vi "TreeMenuUpdate.vi"(4 "error in":errorcluster, 5 "Date?":bool, 6 "stripped path":path, 7 "Tree Refnum":refnum<vi>) -> (0 "error out":errorcluster)   [LabVIEW 2013, in "main.lvlib"]
uses:
  main.lvlib
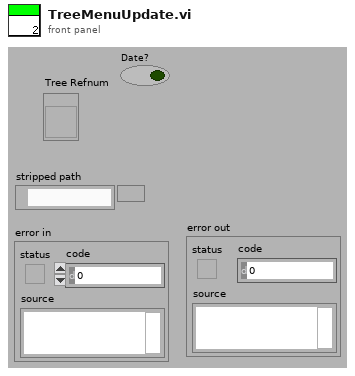
[diagram p1: front panel]
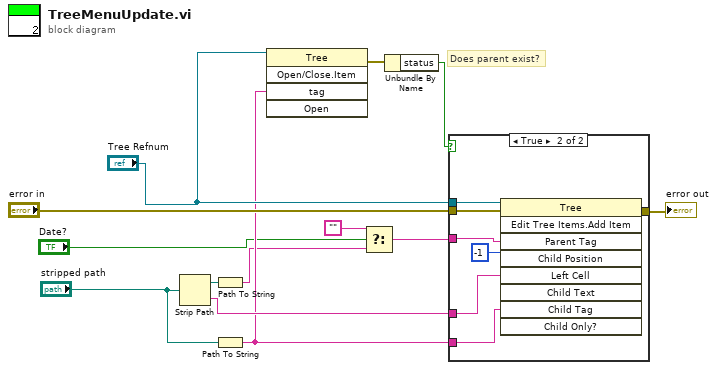
[diagram p0: block diagram]
diagram:
  # "Does parent exist?"
  n1 = Strip Path(path="stripped path") -> (stripped path=w9:path, name=w12:string)
  n2 = Path To String(path=w9) -> (string=w4:string)
  n3 = Path To String(path="stripped path") -> (string=w5:string)
  n4 = invoke class="Tree" method="Open/Close.Item"(reference="Tree Refnum", "tag"=w5) -> (error out=w7:errorcluster)  [unwired: 3 in, 4 out]
  n5 = Select(t="", s="Date?", f=w4) -> (s? t:f=w1:string)
  n6 = Unbundle By Name(w7) -> ("status"=w6:bool)
  n7 = case shown="True" w6 {
    tunnel: [w14 w20] -> w13
    tunnel: w12 -> [_ w19]
    tunnel: w5 -> [_ w18]
    tunnel: "error in" -> [w14 w17]
    tunnel: "Tree Refnum" -> [_ w16]
    tunnel: w1 -> [_ w15]
    frame False {
    }
    frame True {
      n8 = invoke class="Tree" method="Edit Tree Items.Add Item"(reference=w16, error in=w17, "Parent Tag"=w15, "Child Position"=-1, "Left Cell"=w19, "Child Tag"=w18) -> (error out=w20:errorcluster)  [unwired: 3 in, 8 out]
    }
  }
  "error out" <- w13
